vi "Convert 2D Array to Cluster.vi"(8 "error in (no error)":errorcluster, 11 "Array in":string[][](array[string])) -> (0 "error out":errorcluster, 3 "Array out":T1[](array[typedef]))   [LabVIEW 2015, in "Project.lvclass"]
uses:
  Project.lvclass
  FPGA Settings.ctl
  Module/Module/Module Settings.ctl
  Signal/Signal/Signal Settings.ctl
  Signal/Signal/Signal.lvclass
  Module/Module/Module.lvclass
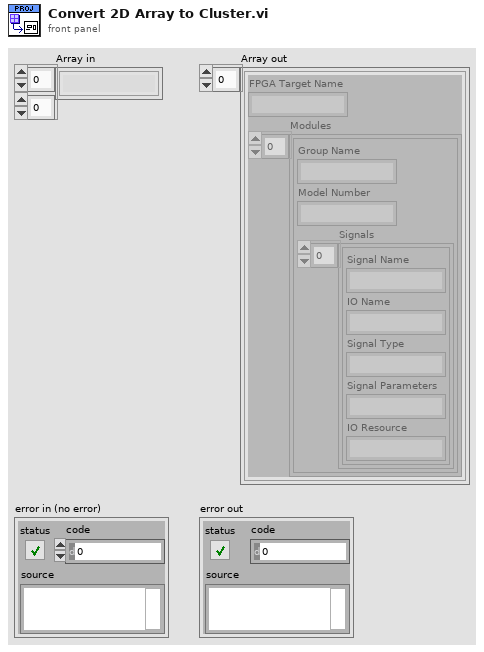
[diagram p1: front panel]
types:
  T1 = typedef "Project.lvclass/FPGA Settings.ctl" = cluster{"FPGA Target Name":string, "Modules":T2[]}
  T2 = typedef "Module.lvclass/Module Settings.ctl" = cluster{"Group Name":string, "Model Number":string, "Signals":T3[]}
  T3 = typedef "Signal.lvclass/Signal Settings.ctl" = cluster{"Signal Name":string, "IO Name":string, "Signal Type":string, "Signal Parameters":string, "IO Resource":string}
  T4 = cluster{"Group Name":string, "Model Number":string, "Signal LUT":variant}
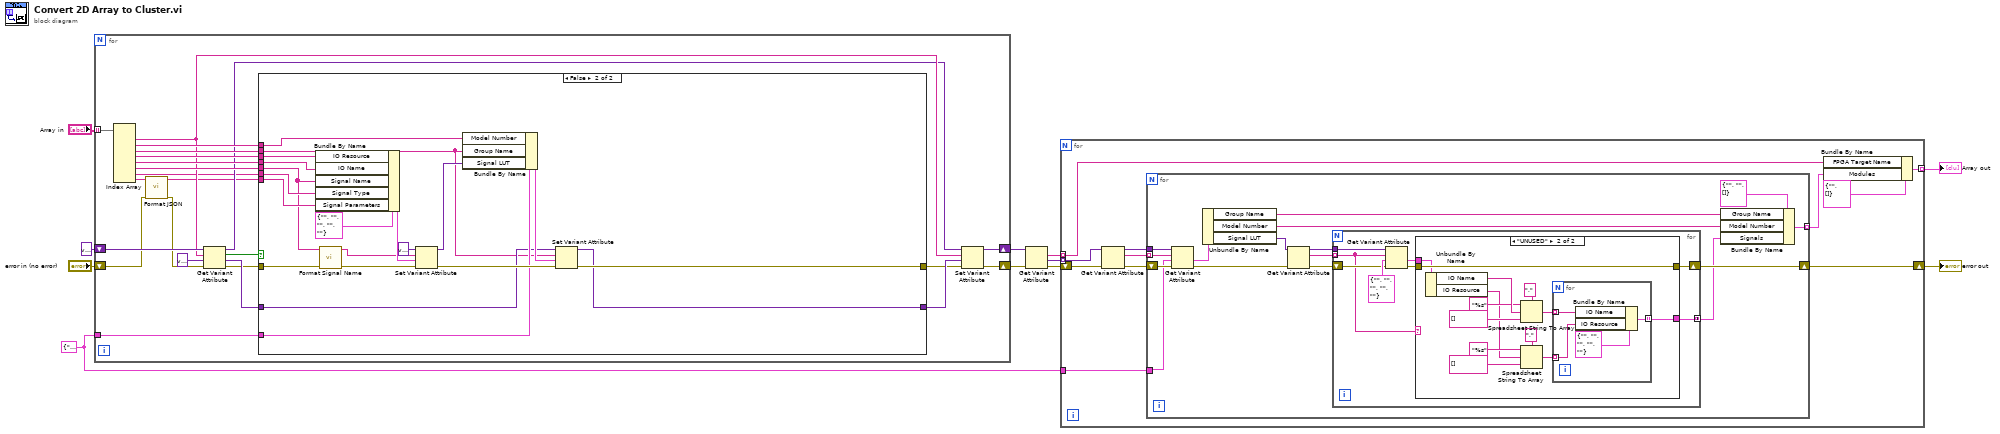
[diagram p0: block diagram]
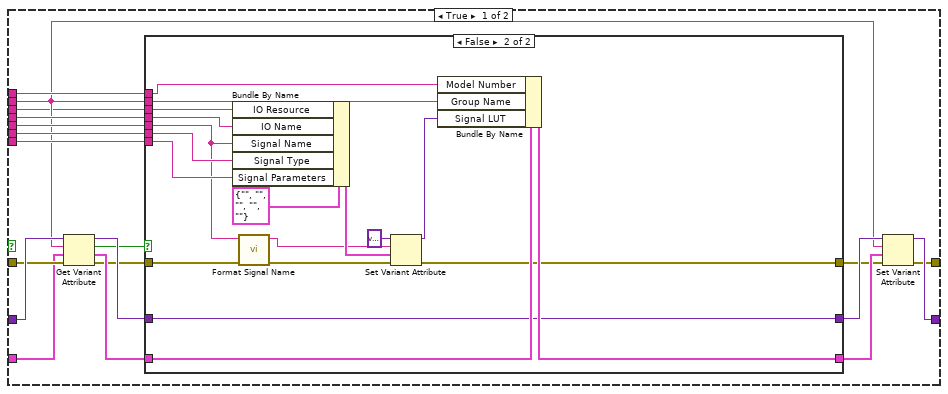
[diagram p2: hidden frame]
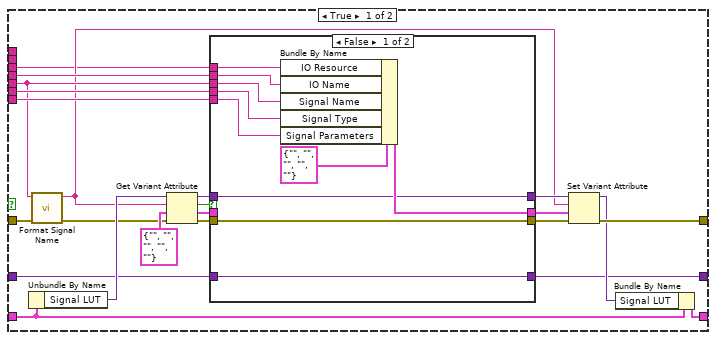
[diagram p3: hidden frame]
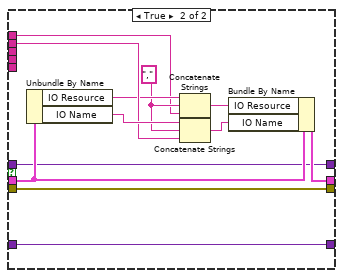
[diagram p4: hidden frame]
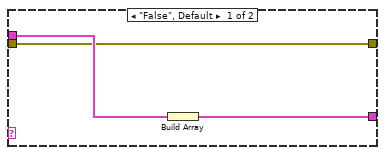
[diagram p5: hidden frame]
diagram:
  w10 = T4 {"Group Name"="", "Model Number"="", "Signal LUT"=variant}
  n1 = for {
    tunnel: "Array in" -> [w33] mode=indexing
    shift-right: [w23] -> w4
    shift-left: variant -> [w34]
    shift-right: [w21] -> w5
    shift-left: "error in (no error)" -> [w16]
    tunnel: w10 -> [w14]
    n2 = Index Array(array=w33) -> (element #1=w19:string, element #2=w25:string, element #3=w26:string, element #4=w27:string, element #5=w28:string, element #6=w29:string, element #7=w12:string, element #8=w13:string)  [unwired: 8 in]
    n3 = call "Format JSON.vi"("error in (no error)"=w16, "String"=w13) -> ("error out"=w15:errorcluster, "String out"=w17:string)  [unwired: 8 in]
    n4 = Get Variant Attribute(Variant=w34, name=w19, default value (empty Variant)=variant ("default value (empty variant)"), error in=w15) -> (duplicate Variant=w18:variant, found=w32:bool, value=w30:variant, error out=w20:errorcluster)
    n5 = case shown="False" w32 {
      tunnel: w30 -> [w53 w121]
      tunnel: w27 -> [w35 w117]
      tunnel: w28 -> [w38 w126]
      tunnel: w29 -> [w39 w125]
      tunnel: w17 -> [w52 w136]
      tunnel: w26 -> [w36 w118]
      tunnel: w25 -> [w37 w119]
      tunnel: [w44 w120] -> w24
      tunnel: [w43 w134] -> w22
      tunnel: w20 -> [w42 w123]
      tunnel: w14 -> [w41 w128]
      tunnel: w12 -> [w40 w127]
      frame True {
        n6 = Get Variant Attribute(Variant=w53, name=w36, default value (empty Variant)=w41, error in=w42) -> (duplicate Variant=w49:variant, found=w47:bool, value=w51:T4, error out=w46:errorcluster)
        n7 = case shown="False" w47 {
          tunnel: w38 -> [w76 w115]
          tunnel: w39 -> [w58 w104]
          tunnel: w40 -> [w75 w114]
          tunnel: w52 -> [w74 w113]
          tunnel: w51 -> [w62 w112]
          tunnel: [w59 w102] -> w50
          tunnel: w49 -> [w70 w102]
          tunnel: [w60 w111] -> w48
          tunnel: w46 -> [w56 w101]
          tunnel: [w64 w107] -> w45
          tunnel: w36 -> [_ w110]
          tunnel: w37 -> [_ w109]
          tunnel: w35 -> [w54 w99]
          frame True {
            n8 = Unbundle By Name(w62) -> ("Signal LUT"=w73:variant)
            n9 = call "Format Signal Name.vi"("error in (no error)"=w56, "String"=w58) -> ("error out"=w55:errorcluster, "String out"=w57:string)  [unwired: 8 in]
            n10 = Get Variant Attribute(Variant=w73, name=w57, default value (empty Variant)=T3 {"Signal Name"="", "IO Name"="", "Signal Type"="", "Signal Parameters"="", "IO Resource"=""}, error in=w55) -> (duplicate Variant=w69:variant, found=w71:bool, value=w68:T3, error out=w67:errorcluster)
            n11 = case shown="False" w71 {
              tunnel: w76 -> [w85 w96]
              tunnel: w75 -> [w84 _]
              tunnel: w74 -> [w83 _]
              tunnel: w58 -> [w82 _]
              tunnel: w70 -> [w79 w98]
              tunnel: w69 -> [w78 w91]
              tunnel: w68 -> [_ w95]
              tunnel: w67 -> [w80 w93]
              tunnel: [w81 w92] -> w66
              tunnel: [w80 w93] -> w65
              tunnel: [w78 w91] -> w63
              tunnel: [w79 w98] -> w59
              tunnel: w54 -> [w77 w88]
              frame False {
                n12 = Bundle By Name(cluster=T3 {"Signal Name"="", "IO Name"="", "Signal Type"="", "Signal Parameters"="", "IO Resource"=""}, "IO Resource"=w77, "IO Name"=w85, "Signal Name"=w82, "Signal Type"=w84, "Signal Parameters"=w83) -> (w81:T3)
              }
              frame True {
                w89 = "," ("string")
                n13 = Unbundle By Name(w95) -> ("IO Resource"=w90:string, "IO Name"=w97:string)
                n14 = Concatenate Strings(w90, w89, w88) -> (w87:string)
                n15 = Concatenate Strings(w97, w89, w96) -> (w94:string)
                n16 = Bundle By Name(cluster=w95, "IO Resource"=w87, "IO Name"=w94) -> (w92:T3)
              }
            }
            n17 = Set Variant Attribute(Variant=w63, name=w57, value=w66, error in=w65) -> (Variant out=w61:variant, error out=w64:errorcluster)  [unwired: 1 out]
            n18 = Bundle By Name(cluster=w62, "Signal LUT"=w61) -> (w60:T4)
          }
          frame False {
            n19 = Bundle By Name(cluster=T3 {"Signal Name"="", "IO Name"="", "Signal Type"="", "Signal Parameters"="", "IO Resource"=""}, "IO Resource"=w99, "IO Name"=w115, "Signal Name"=w104, "Signal Type"=w114, "Signal Parameters"=w113) -> (w108:T3)
            n20 = call "Format Signal Name.vi"("error in (no error)"=w101, "String"=w104) -> ("error out"=w100:errorcluster, "String out"=w103:string)  [unwired: 8 in]
            n21 = Set Variant Attribute(Variant=variant ("variant"), name=w103, value=w108, error in=w100) -> (Variant out=w105:variant, error out=w107:errorcluster)  [unwired: 1 out]
            n22 = Bundle By Name(cluster=w112, "Model Number"=w109, "Group Name"=w110, "Signal LUT"=w105) -> (w111:T4)
          }
        }
        n23 = Set Variant Attribute(Variant=w50, name=w36, value=w48, error in=w45) -> (Variant out=w44:variant, error out=w43:errorcluster)  [unwired: 1 out]
      }
      frame False {
        n24 = Bundle By Name(cluster=T3 {"Signal Name"="", "IO Name"="", "Signal Type"="", "Signal Parameters"="", "IO Resource"=""}, "IO Resource"=w117, "IO Name"=w126, "Signal Name"=w125, "Signal Type"=w127, "Signal Parameters"=w136) -> (w132:T3)
        n25 = call "Format Signal Name.vi"("error in (no error)"=w123, "String"=w125) -> ("error out"=w122:errorcluster, "String out"=w124:string)  [unwired: 8 in]
        n26 = Set Variant Attribute(Variant=variant ("variant"), name=w124, value=w132, error in=w122) -> (Variant out=w130:variant, error out=w129:errorcluster)  [unwired: 1 out]
        n27 = Bundle By Name(cluster=w128, "Model Number"=w119, "Group Name"=w118, "Signal LUT"=w130) -> (w135:T4)
        n28 = Set Variant Attribute(Variant=w121, name=w118, value=w135, error in=w129) -> (Variant out=w120:variant, error out=w134:errorcluster)  [unwired: 1 out]
      }
    }
    n29 = Set Variant Attribute(Variant=w18, name=w19, value=w24, error in=w22) -> (Variant out=w23:variant, error out=w21:errorcluster)  [unwired: 1 out]
  }
  n30 = Get Variant Attribute(Variant=w4, error in=w5) -> (names=w6:string[], values=w7:variant[], error out=w8:errorcluster)  [unwired: 2 in, 1 out]
  n31 = for {
    tunnel: w6 -> [w146] mode=indexing
    tunnel: w7 -> [w145] mode=indexing
    shift-right: [w141] -> w9
    shift-left: w8 -> [w144]
    tunnel: [w140] -> w11 mode=indexing
    tunnel: w10 -> [w138]
    n32 = Get Variant Attribute(Variant=w145, error in=w144) -> (duplicate Variant=w139:variant, names=w142:string[], error out=w143:errorcluster)  [unwired: 2 in, 1 out]
    n33 = for {
      shift-right: [w150] -> w141
      shift-left: w143 -> [w163]
      tunnel: w142 -> [w162] mode=indexing
      tunnel: w139 -> [w160]
      tunnel: w138 -> [w159]
      tunnel: [w148] -> w137 mode=indexing
      n34 = Get Variant Attribute(Variant=w160, name=w162, default value (empty Variant)=w159, error in=w163) -> (value=w161:T4, error out=w154:errorcluster)  [unwired: 2 out]
      n35 = Unbundle By Name(w161) -> ("Group Name"=w157:string, "Model Number"=w156:string, "Signal LUT"=w155:variant)
      n36 = Get Variant Attribute(Variant=w155, error in=w154) -> (duplicate Variant=w153:variant, names=w152:string[], error out=w151:errorcluster)  [unwired: 2 in, 1 out]
      n37 = for {
        tunnel: w153 -> [w171]
        tunnel: w152 -> [w164] mode=indexing
        shift-right: [w166] -> w150
        shift-left: w151 -> [w169]
        tunnel: [w167] -> w149 mode=concatenating
        n38 = Get Variant Attribute(Variant=w171, name=w164, default value (empty Variant)=T3 {"Signal Name"="", "IO Name"="", "Signal Type"="", "Signal Parameters"="", "IO Resource"=""}, error in=w169) -> (value=w168:T3, error out=w165:errorcluster)  [unwired: 2 out]
        n39 = case shown="\"UNUSED\"" w164 {
          tunnel: w168 -> [w174 w181]
          tunnel: [w173 w180] -> w167
          tunnel: [w172 w187] -> w166
          tunnel: w165 -> [w172 w187]
          frame "False", Default {
            n40 = Build Array(w174) -> (w173:T3[])
          }
          frame "UNUSED" {
            n41 = Unbundle By Name(w181) -> ("IO Name"=w186:string, "IO Resource"=w176:string)
            n42 = Spreadsheet String To Array(delimiter (Tab)=",", format string="%s", spreadsheet string=w186, array type (2D Dbl)=string[] []) -> (array=w182:string[])
            n43 = Spreadsheet String To Array(delimiter (Tab)=",", format string="%s", spreadsheet string=w176, array type (2D Dbl)=string[] []) -> (array=w175:string[])
            n44 = for {
              tunnel: w182 -> [w190] mode=indexing
              tunnel: [w189] -> w180 mode=indexing
              tunnel: w175 -> [w188] mode=indexing
              n45 = Bundle By Name(cluster=T3 {"Signal Name"="", "IO Name"="", "Signal Type"="", "Signal Parameters"="", "IO Resource"=""}, "IO Name"=w190, "IO Resource"=w188) -> (w189:T3)
            }
          }
        }
      }
      n46 = Bundle By Name(cluster=T2 {"Group Name"="", "Model Number"="", "Signals"=[]}, "Group Name"=w157, "Model Number"=w156, "Signals"=w149) -> (w148:T2)
    }
    n47 = Bundle By Name(cluster=T1 {"FPGA Target Name"="", "Modules"=[]} ("FPGA Settings"), "FPGA Target Name"=w146, "Modules"=w137) -> (w140:T1)
  }
  "Array out" <- w11
  "error out" <- w9
